vi "CIF Template UI.vi"() -> ()   [LabVIEW 2021, in "CIF Template UI.lvlib"]
uses:
  CIF Template UI.lvlib
  CIF-LVCore/src/CIFCore/Common/Typedef/gRPC Reported Plugin Status.ctl
  CIF-LVCore/src/CIFCore/Common/Typedef/Plugin State.ctl
  CIF-LVCore/src/CIFCore/Common/Typedef/Timing Statistics.ctl
  CIF-LVCore/src/CIFCore/Common/Typedef/Timing Stats Base.ctl
  CIF-LVCore/src/CIFCore/Common/Typedef/FIFO Statistics.ctl
  CIF-LVCore/src/CIFCore/Common/Typedef/Simple Error.ctl
  CIF-LVCore/src/CIFCore/Common/Typedef/Monitor Doubles.ctl
  CIF-LVCore/src/CIFCore/Common/Typedef/Monitor U64.ctl
  CIF-LVCore/src/CIFCore/Common/Typedef/Monitor I64.ctl
  Instrument Studio/PluginSDK/Plugin Events Enum.ctl
  CIF-LVCore/src/CIFCore/Grpc/CIFCoreChannel_client/RPC Messages/cif_channelcore_ForceChannel.ctl
  <vilib>/gRPC/LabVIEW gRPC Library/Client API/Close Client.vi
  Instrument Studio/PluginSDK/Plugin Session.lvclass
  Instrument Studio/PluginSDK/InstrumentStudio Plugin SDK.lvlib
  CIF-LVCore/src/CIFCore/Grpc/CIFCoreWrapper/CIFCoreWrapper.lvlib
  CIF-LVCore/src/CIFUI/CIF_UI.lvclass
  CIF-LVCore/src/CIFCore/Grpc/CIFCoreChannel_client/CIFCoreChannel_client.lvlib
  Grpc/Template_wrapper/TemplateWrapper.lvlib
  CIF-LVCore/src/CIFCore/Common/CIFCoreCommon.lvlib
panel:
  in  "Force":bool
  out "Current Config":string
  in  "New Config":string
  in  "Unload":bool
  out "Node Status":T1 {"Monitor Doubles"."4" format="%#_9g"; "Monitor Doubles"."3" format="%#_9g"; "Monitor Doubles"."2" format="%#_9g"; "Monitor Doubles"."1" format="%#_9g"}
  in  "Refresh Button":bool
  in  "Pause":bool
  in  "Start":bool
  out "Connected":bool
  in  "Connect":bool
  in  "stop":bool
  in  "address":string="192.168.1.160"
  out "local error":errorcluster
  in  "Clear Local":bool
  in  "Channels":string(tree)
  in  "Update Config":bool
  in  "Force Channel":T10
  in  "Session Id":u64
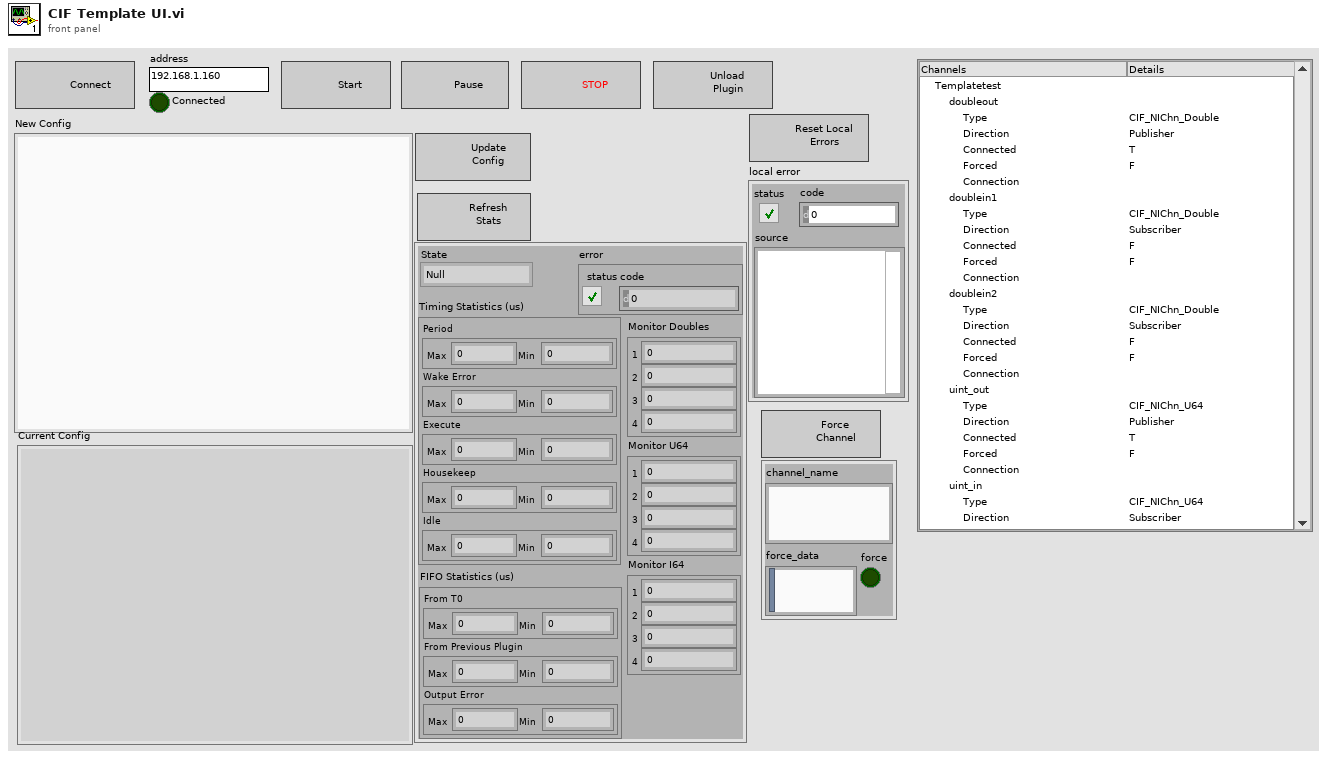
[diagram p1: front panel]
types:
  T1 = typedef "CIFCoreCommon.lvlib/gRPC Reported Plugin Status.ctl" = cluster{"State":T2, "Timing Statistics (us)":T3, "FIFO Statistics (us)":T5, "error":T6, "Monitor Doubles":T7, "Monitor U64":T8, "Monitor I64":T9}
  T2 = typedef "CIFCoreCommon.lvlib/Plugin State.ctl" = enum32{"Null", "Creating", "Listening", "Running", "CleaningUp", "Destroying"}
  T3 = typedef "CIFCoreCommon.lvlib/Timing Statistics.ctl" = cluster{"Period":T4, "Wake Error":T4, "Execute":T4, "Housekeep":T4, "Idle":T4}
  T4 = typedef "CIFCoreCommon.lvlib/Timing Stats Base.ctl" = cluster{"Max":i32, "Min":i32}
  T5 = typedef "CIFCoreCommon.lvlib/FIFO Statistics.ctl" = cluster{"From T0":T4, "From Previous Plugin":T4, "Output Error":T4}
  T6 = typedef "CIFCoreCommon.lvlib/Simple Error.ctl" = cluster{"status":bool, "code":i32}
  T7 = typedef "CIFCoreCommon.lvlib/Monitor Doubles.ctl" = cluster{"1":dbl, "2":dbl, "3":dbl, "4":dbl}
  T8 = typedef "CIFCoreCommon.lvlib/Monitor U64.ctl" = cluster{"1":u64, "2":u64, "3":u64, "4":u64}
  T9 = typedef "CIFCoreCommon.lvlib/Monitor I64.ctl" = cluster{"1":i64, "2":i64, "3":i64, "4":i64}
  T10 = cluster{"channel_name":string, "force":bool, "force_data":string}
  T11 = typedef "InstrumentStudio Plugin SDK.lvlib/Plugin Events Enum.ctl" = enum32{"Shutdown", "Project Saved", "Stop All Outputs", "Generic Message", "Active Pin Map Changed", "Selected Sites Changed"}
  T12 = typedef "InstrumentStudio Plugin SDK.lvlib/Event Registration Refnum.ctl" = refnum<event-registration>
  T13 = typedef "CIFCoreChannel_client.lvlib/cif_channelcore_ForceChannel.ctl" = cluster{"channel_name":string, "force":bool, "force_data":u8[]}
  T14 = typedef "CIFCoreChannel_client.lvlib/cif_channelcore_Direction.ctl" = enum32{"PUBLISHER", "SUBSCRIBER"}
  T15 = cluster{"name":string, "direction":T14, "type":string, "custom_config":u8[], "connected":bool, "connected_name":string, "forced":bool}[]
  T16 = typedef "grpc-lvsupport-release.lvlib/grpcId.ctl" = u64
  T17 = cluster{"name":string, "direction":T14, "type":string, "custom_config":u8[], "connected":bool, "connected_name":string, "forced":bool}[][]
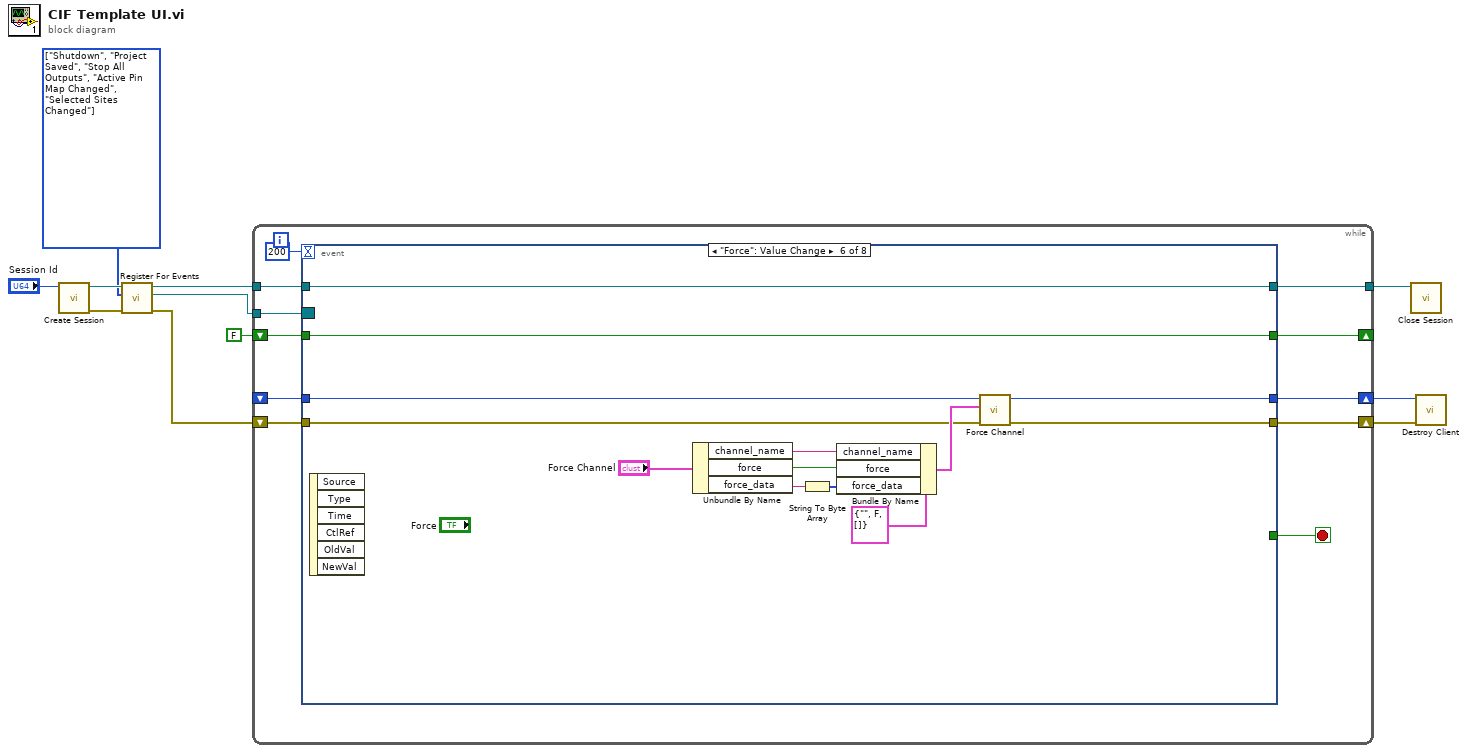
[diagram p0: block diagram]
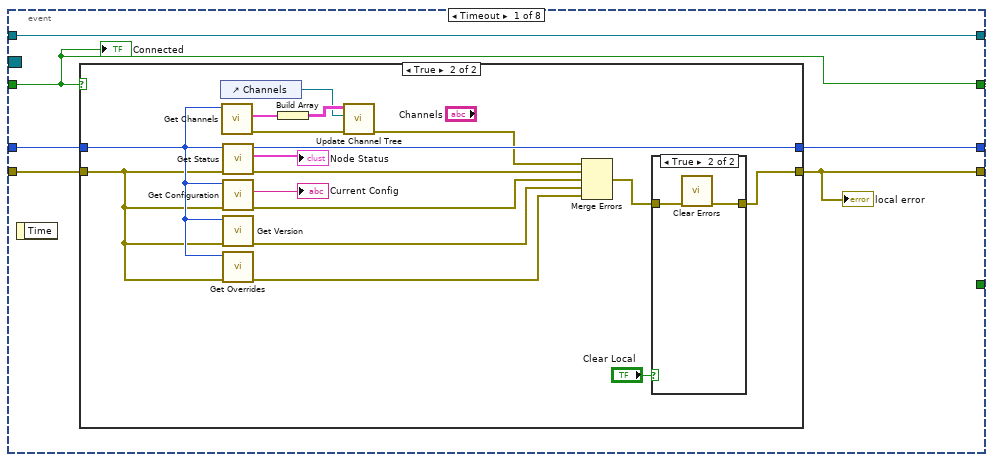
[diagram p2: hidden frame]
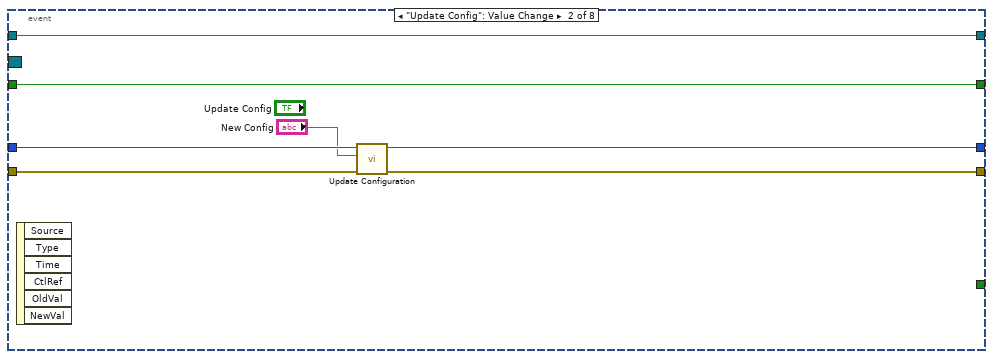
[diagram p5: hidden frame]
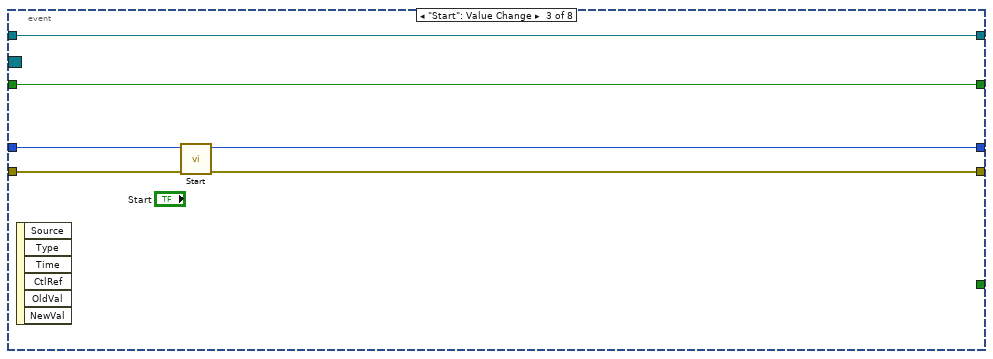
[diagram p6: hidden frame]
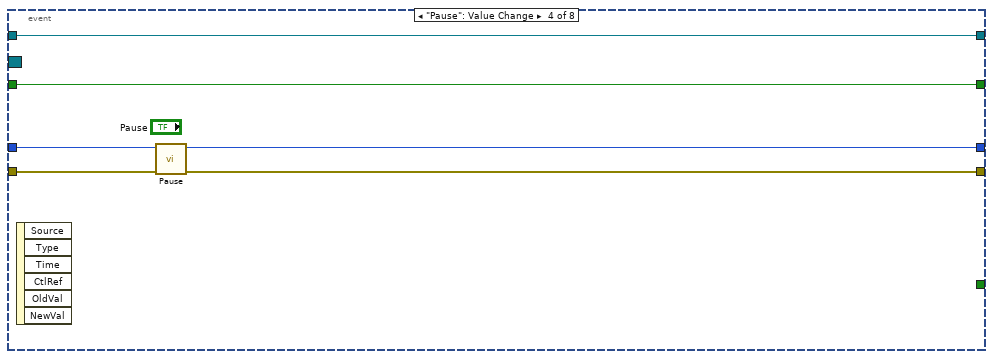
[diagram p7: hidden frame]
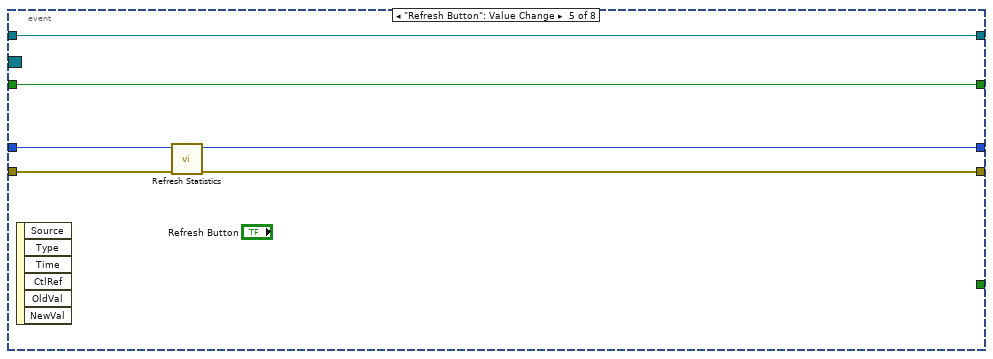
[diagram p8: hidden frame]
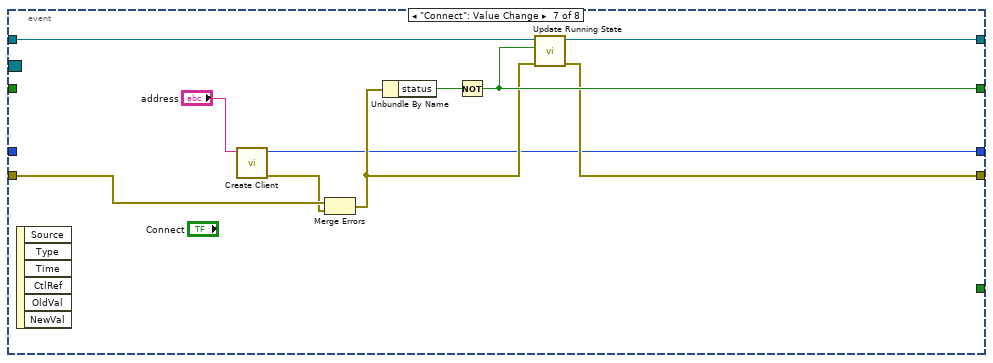
[diagram p9: hidden frame]
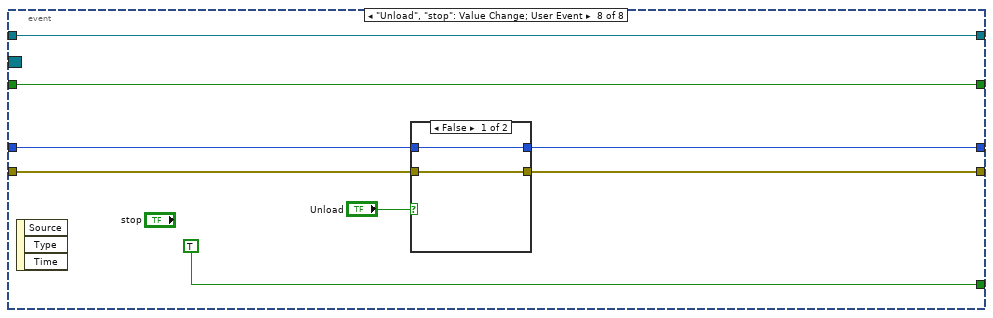
[diagram p10: hidden frame]
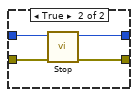
[diagram p11: hidden frame]
diagram:
  w7 = T11[] [enum."Shutdown", enum."Project Saved", enum."Stop All Outputs", enum."Active Pin Map Changed", enum."Selected Sites Changed"] items=["Shutdown", "Project Saved", "Stop All Outputs", "Generic Message", "Active Pin Map Changed", "Selected Sites Changed"] ("Events To Register")
  n1 = call "Create Session.vi"("Session Id"="Session Id") -> ("error out"=w4:errorcluster, "Session out"=w10:refnum<class "Plugin Session.lvclass">)  [unwired: 6 in, 3 out]
  n2 = call "Register For Events.vi"("error in (no error)"=w4, "Events To Register"=w7, "Session in"=w10) -> ("error out"=w1:errorcluster, "Event Refnum"=w6:T12, "Session out"=w9:refnum<class "Plugin Session.lvclass">)  [unwired: 6 in]
  n3 = while {
    tunnel: w9 -> [w21]
    tunnel: [w20] -> w8
    tunnel: w6 -> [w19]
    shift-right: [w14] -> w2
    shift-left: _ -> [w17]
    shift-right: [w12] -> _
    shift-left: FALSE -> [w13]
    shift-right: [w15] -> w3
    shift-left: w1 -> [w16]
    stop <- w18 stop-if-true
    n4 = event shown="[5] \"Force\": Value Change" {
      selector: w19 -> [_ _ _ _ _ _ _ _]
      dyn-events: _ -> [_ _ _ _ _ _ _ _]
      timeout: 200 -> [_ _ _ _ _ _ _ _]
      tunnel: w21 -> [w28 w52 w58 w64 w70 w88 w96 w105]
      tunnel: [w28 w52 w58 w64 w70 w88 w95 w105] -> w20
      tunnel: [_ _ _ _ _ _ _ TRUE] -> w18
      tunnel: w17 -> [w24 w57 w63 w69 w75 w79 _ w103]
      tunnel: w16 -> [w27 w56 w62 w68 w74 w76 w98 w102]
      tunnel: [w26 w54 w60 w66 w72 w77 w93 w100] -> w15
      tunnel: [w23 w55 w61 w67 w73 w78 w90 w101] -> w14
      tunnel: w13 -> [w25 w53 w59 w65 w71 w87 _ w104]
      tunnel: [w25 w53 w59 w65 w71 w87 w94 w104] -> w12
      event Timeout {
        n5 = event-data() -> ()  [unwired: 1 in, 1 out]
        n6 = case shown="True" w25 {
          tunnel: w27 -> [w30 w31]
          tunnel: [w30 w47] -> w26
          tunnel: w24 -> [w29 w32]
          tunnel: [w29 w44] -> w23
          frame False {
          }
          frame True {
            n7 = control-ref of="Channels"() -> (w33:refnum<vi>)
            n8 = call "Get Channels.vi"("gRPC ID"=w32) -> ("error out"=w35:errorcluster, "Channels"=w37:T15)  [unwired: 8 in, 1 out]
            n9 = call "Get Status.vi"("error in"=w31, "gRPC ID"=w32) -> ("error out"=w43:errorcluster, "Node Status"=→"Node Status":T1, "gRPC ID out"=w44:T16)  [unwired: 7 in]
            n10 = call "Get Configuration.vi"("error in"=w31, "gRPC ID"=w32) -> ("error out"=w42:errorcluster, "JSON Configuration"=→"Current Config":string)  [unwired: 7 in, 1 out]
            n11 = call "Get Version.vi"("error in"=w31, "gRPC ID"=w32) -> ("error out"=w40:errorcluster)  [unwired: 7 in, 2 out]
            n12 = call "Get Overrides.vi"("error in"=w31, "gRPC ID"=w32) -> ("error out"=w41:errorcluster)  [unwired: 7 in, 2 out]
            n13 = Build Array(w37) -> (w36:T17)
            n14 = call "Update Channel Tree.vi"("error in (no error)"=w35, "Channnel Tree ref in"=w33, "Channels"=w36) -> ("error out"=w34:errorcluster)  [unwired: 8 in]
            n15 = Merge Errors(w34, w43, w42, w40, w41) -> (w45:errorcluster)
            n16 = case shown="True" "Clear Local" {
              tunnel: w45 -> [w48 w50]
              tunnel: [w48 w49] -> w47
              frame False {
              }
              frame True {
                n17 = call <vilib>:"Clear Errors.vi"("error in (no error)"=w50) -> ("error out"=w49:errorcluster)  [unwired: 5 in, 1 out]
              }
            }
          }
        }
        "local error" <- w26
        "Connected" <- w25
      }
      event "Update Config": Value Change {
        n18 = event-data() -> ()  [unwired: 1 in, 6 out]
        n19 = call "Update Configuration.vi"("error in"=w56, "JSON Configuration"="New Config", "gRPC ID"=w57) -> ("error out"=w54:errorcluster, "gRPC ID out"=w55:T16)  [unwired: 7 in]
      }
      event "Start": Value Change {
        n20 = event-data() -> ()  [unwired: 1 in, 6 out]
        n21 = call "Start.vi"("error in"=w62, "gRPC ID"=w63) -> ("error out"=w60:errorcluster, "gRPC ID out"=w61:T16)  [unwired: 8 in]
      }
      event "Pause": Value Change {
        n22 = event-data() -> ()  [unwired: 1 in, 6 out]
        n23 = call "Pause.vi"("error in"=w68, "gRPC ID"=w69) -> ("error out"=w66:errorcluster, "gRPC ID out"=w67:T16)  [unwired: 8 in]
      }
      event "Refresh Button": Value Change {
        n24 = event-data() -> ()  [unwired: 1 in, 6 out]
        n25 = call "Refresh Statistics.vi"("error in"=w74, "gRPC ID"=w75) -> ("error out"=w72:errorcluster, "gRPC ID out"=w73:T16)  [unwired: 8 in]
      }
      event "Force": Value Change {
        n26 = event-data() -> ()  [unwired: 1 in, 6 out]
        n27 = Unbundle By Name("Force Channel") -> ("channel_name"=w86:string, "force"=w83:bool, "force_data"=w81:string)
        n28 = String To Byte Array(string=w81) -> (unsigned byte array=w82:u8[])
        n29 = Bundle By Name(cluster=T13 {"channel_name"="", "force"=FALSE, "force_data"=[]} ("Force Channel"), "channel_name"=w86, "force"=w83, "force_data"=w82) -> (w84:T13)
        n30 = call "Force Channel.vi"("error in"=w76, "Force Channel"=w84, "gRPC ID"=w79) -> ("error out"=w77:errorcluster, "gRPC ID out"=w78:T16)  [unwired: 7 in]
      }
      event "Connect": Value Change {
        n31 = event-data() -> ()  [unwired: 1 in, 6 out]
        n32 = call "Create Client.vi"("address"="address") -> ("error out"=w89:errorcluster, "gRPC ID Out"=w90:T16)  [unwired: 9 in]
        n33 = Merge Errors(w98, w89) -> (w92:errorcluster)
        n34 = Unbundle By Name(w92) -> ("status"=w97:bool)
        n35 = Not(x=w97) -> (.not. x?=w94:bool)
        n36 = call "Update Running State.vi"("error in (no error)"=w92, "Is Running"=w94, "Plugin Session in"=w96) -> ("error out"=w93:errorcluster, "Plugin Session out"=w95:refnum<class "Plugin Session.lvclass">)  [unwired: 7 in]
      }
      event "Unload", "stop": Value Change; User Event {
        n37 = event-data() -> ()  [unwired: 1 in, 3 out]
        n38 = case shown="False" "Unload" {
          tunnel: w103 -> [w108 w112]
          tunnel: w102 -> [w107 w111]
          tunnel: [w108 w110] -> w101
          tunnel: [w107 w109] -> w100
          frame False {
          }
          frame True {
            n39 = call "Stop.vi"("error in"=w111, "gRPC ID"=w112) -> ("error out"=w109:errorcluster, "gRPC ID out"=w110:T16)  [unwired: 8 in]
          }
        }
      }
    }
  }
  n40 = call "Close Session.vi"("Session in"=w8) -> ()  [unwired: 10 in, 1 out]
  n41 = call "Destroy Client.vi"("error in"=w3, "gRPC ID"=w2) -> ()  [unwired: 9 in, 1 out]
